vi "CCWorklistSCUSequenceItems.vi"(8 "error in (no error)":errorcluster, 9 "Array in":string[](array[string]), 10 "new reference":refnum<k24>, 11 ".NET Refnum in":refnum<k24>) -> (0 "error out":errorcluster, 3 "Array out":string[](array[string]))   [LabVIEW 2013, in "main.lvlib" / "ClearCanvasLibrary.lvlib"]
uses:
  ClearCanvasLibrary.lvlib
  C:/Users/Simon/SkyDrive/LabView/2013/DM2020/DICOM/ClearCanvasNewBuild/ClearCanvas.Dicom.dll
  ClearCanvasNewBuild/ClearCanvas.Dicom.dll
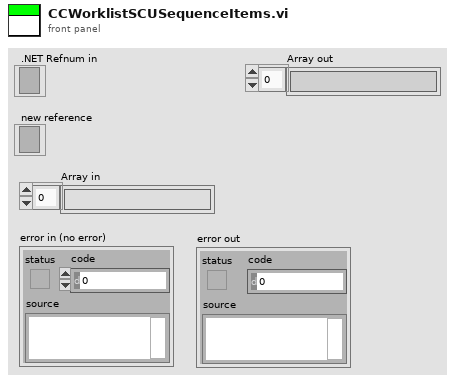
[diagram p1: front panel]
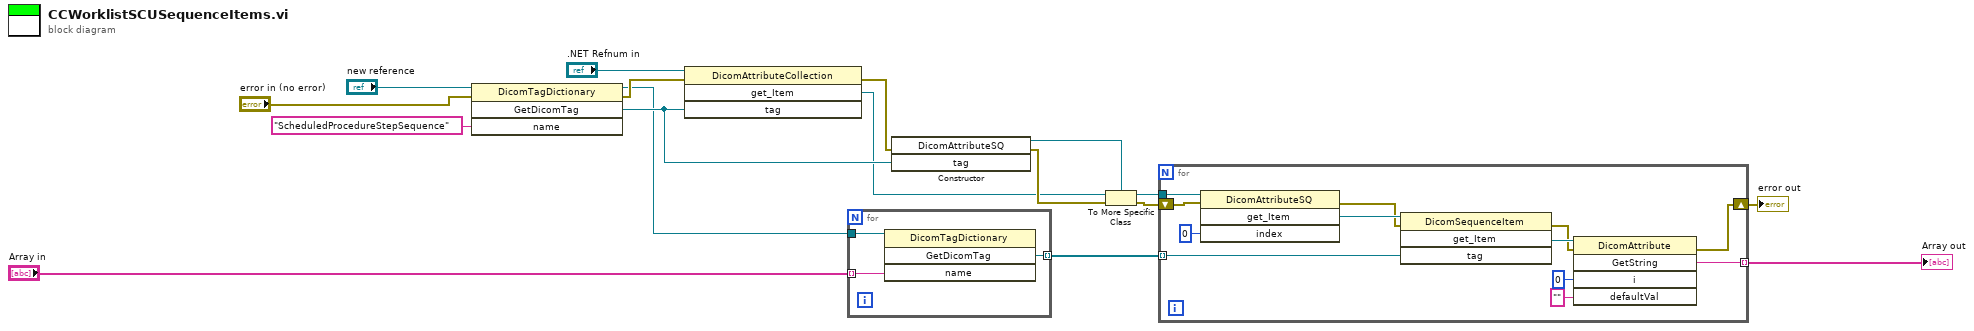
[diagram p0: block diagram]
diagram:
  n1 = invoke class="DicomTagDictionary" method="GetDicomTag"(reference="new reference", error in="error in (no error)", "name"="ScheduledProcedureStepSequence") -> (reference out=w6:refnum<k24>, error out=w14:errorcluster, "GetDicomTag"=w10:refnum<k24>)  [unwired: 1 in, 1 out]
  n2 = invoke class="DicomAttributeCollection" method="get_Item"(reference=".NET Refnum in", error in=w14, "tag"=w10) -> (error out=w15:errorcluster, "get_Item"=w9:refnum<k24>)  [unwired: 1 in, 2 out]
  n3 = for {
    tunnel: w6 -> [w20]
    tunnel: "Array in" -> [w19] mode=indexing
    tunnel: [w18] -> w12 mode=indexing
    n4 = invoke class="DicomTagDictionary" method="GetDicomTag"(reference=w20, "name"=w19) -> ("GetDicomTag"=w18:refnum<k24>)  [unwired: 2 in, 3 out]
  }
  n5 = constructor class="DicomAttributeSQ"(error in=w15, "tag"=w10) -> (reference out=w11:refnum<k24>, error out=w16:errorcluster)  [unwired: 2 in, 2 out]
  n6 = To More Specific Class(target class=w11, reference=w9, error in=w16) -> (specific class reference=w8:refnum<k24>, error out=w17:errorcluster)
  n7 = for {
    tunnel: w8 -> [w32]
    tunnel: w12 -> [w29] mode=indexing
    tunnel: [w25] -> w13 mode=indexing
    shift-right: [w23] -> w1
    shift-left: w17 -> [w24]
    n8 = invoke class="DicomAttributeSQ" method="get_Item"(reference=w32, error in=w24, "index"=0) -> (error out=w21:errorcluster, "get_Item"=w31:refnum<k24>)  [unwired: 1 in, 2 out]
    n9 = invoke class="DicomSequenceItem" method="get_Item"(reference=w31, error in=w21, "tag"=w29) -> (error out=w22:errorcluster, "get_Item"=w28:refnum<k24>)  [unwired: 1 in, 2 out]
    n10 = invoke class="DicomAttribute" method="GetString"(reference=w28, error in=w22, "i"=0, "defaultVal"="") -> (error out=w23:errorcluster, "GetString"=w25:string)  [unwired: 1 in, 3 out]
  }
  "Array out" <- w13
  "error out" <- w1
